vi "add_string.vi"   [LabVIEW 2010]
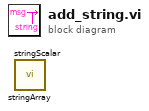
[diagram p0: block diagram]
diagram:
  n1 = call <userlib>:"stringArray.vi"() -> ()  [unwired: 5 in, 1 out]
  n2 = call <userlib>:"stringScalar.vi"() -> ()  [unwired: 5 in, 1 out]
